vi "LED Loop.vi"   [LabVIEW 2016]
uses:
  <vilib>/Rock Robotics/WPI/DriverStation/WPI_DriverStationRobotMode2.ctl
  Common Code/Shooter Commands.ctl
  Robot Code/Robot Global Data.vi
types:
  T1 = typedef "Shooter Commands.ctl" = enum16{"Idle ", "Warmup ", "Shoot"}
  T2 = typedef "WPI_DriverStationRobotMode2.ctl" = enum16{"Autonomous Disabled", "Autonomous Enabled", "Teleop Disabled", "Teleop Enabled", "Disconnected", "Finish", "Test Disabled", "Test Enabled", "Emergency Stopped"}
  T3 = typedef "Shooter Control Cluster'.ctl" = cluster{"Shooter Modes":T4, "Shooter Commands":T1, "manUEL Control Cluster":T5, "Shot Type":T6}
  T4 = typedef "Shooter Modes.ctl" = enum16{"Auto", "Manual"}
  T5 = typedef "Manual Shoot Cluster.ctl" = cluster{"Shot RPM":dbl, "Wait Time":dbl, "da HOOD?":bool}
  T6 = typedef "Shot Type.ctl" = enum16{"Vision Shot", "Dist Shot", "Key Shot"}
  T7 = typedef "Climb Command Cluster.ctl" = cluster{"Go Up":bool}
  T8 = typedef "WPI_AOChannelDevRef.ctl" = cluster{"DevStatus":errorcluster, "AO Channel":T9}
  T9 = typedef "WPI_AnalogOutputChannel.ctl" = enum8{"AO MXP 0", "AO MXP 1", "Invalid"}
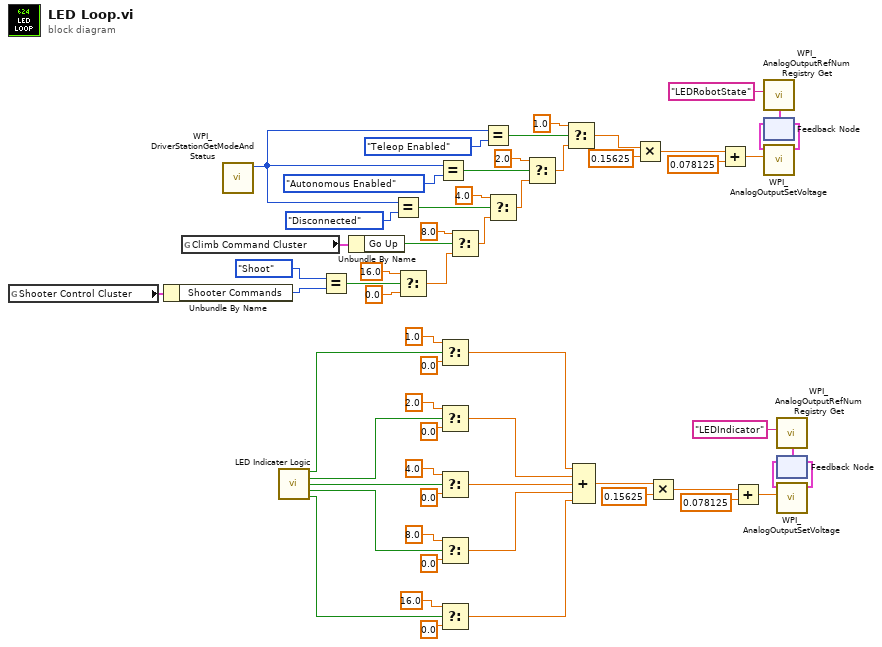
[diagram p0: block diagram]
diagram:
  n1 = global read "Robot Global Data.vi" "Shooter Control Cluster"() -> (w20:T3)
  n2 = Unbundle By Name(w20) -> ("Shooter Commands"=w18:T1)
  n3 = global read "Robot Global Data.vi" "Climb Command Cluster"() -> (w23:T7)
  n4 = call <vilib>:"WPI_DriverStationGetModeAndStatus.vi"() -> ("Robot Mode"=w27:T2)  [unwired: 10 in, 1 out]
  n5 = call "LED Indicater Logic.vi"() -> ("Read4Gear"=w61:bool, "Traction"=w58:bool, "Intake"=w57:bool, "Brakes"=w59:bool, "Hood Up"=w60:bool)  [unwired: 11 in]
  n6 = Equal?(x=Shooter_Commands."Shoot" ("Shooter Commands"), y=w18) -> (x = y?=w16:bool)
  n7 = Unbundle By Name(w23) -> ("Go Up"=w21:bool)
  n8 = Equal?(x=w27, y=WPI_DriverStationRobotMode2."Disconnected" ("Robot Mode")) -> (x = y?=w30:bool)
  n9 = Select(t=16.0, s=w16, f=0.0) -> (s? t:f=w17:dbl)
  n10 = Equal?(x=w27, y=WPI_DriverStationRobotMode2."Autonomous Enabled" ("Robot Mode")) -> (x = y?=w29:bool)
  n11 = Select(t=1.0, s=w61, f=0.0) -> (s? t:f=w46:dbl)
  n12 = Select(t=2.0, s=w58, f=0.0) -> (s? t:f=w45:dbl)
  n13 = Select(t=4.0, s=w57, f=0.0) -> (s? t:f=w44:dbl)
  n14 = Select(t=8.0, s=w59, f=0.0) -> (s? t:f=w43:dbl)
  n15 = Select(t=16.0, s=w60, f=0.0) -> (s? t:f=w42:dbl)
  n16 = Select(t=8.0, s=w21, f=w17) -> (s? t:f=w22:dbl)
  n17 = Equal?(x=w27, y=WPI_DriverStationRobotMode2."Teleop Enabled" ("Robot Mode")) -> (x = y?=w28:bool)
  n18 = Select(t=4.0, s=w30, f=w22) -> (s? t:f=w32:dbl)
  n19 = Select(t=2.0, s=w29, f=w32) -> (s? t:f=w31:dbl)
  n20 = Select(t=1.0, s=w28, f=w31) -> (s? t:f=w6:dbl)
  n21 = Compound Arithmetic op=ADD(w46, w45, w44, w43, w42) -> (w41:dbl)
  n22 = Multiply(x=w6, y=0.15625) -> (x*y=w8:dbl)
  n23 = Multiply(x=w41, y=0.15625) -> (x*y=w39:dbl)
  n24 = Add(x=w8, y=0.078125) -> (x+y=w1:dbl)
  n25 = Add(x=w39, y=0.078125) -> (x+y=w34:dbl)
  n26 = call <vilib>:"WPI_AnalogOutputRefNum Registry Get.vi"("refnum name"="LEDRobotState") -> ("AODeviceRef"=w4:T8)  [unwired: 9 in, 1 out]
  n27 = feedback #1(w4) -> (w3:T8)
  n28 = call <vilib>:"WPI_AnalogOutputSetVoltage.vi"("Voltage"=w1, "AODeviceRef"=w3) -> ("AODeviceRef"=w2:T8)  [unwired: 8 in, 1 out]
  n29 = feedback-in #1(w2) -> ()
  n30 = call <vilib>:"WPI_AnalogOutputRefNum Registry Get.vi"("refnum name"="LEDIndicator") -> ("AODeviceRef"=w35:T8)  [unwired: 9 in, 1 out]
  n31 = feedback #2(w35) -> (w36:T8)
  n32 = call <vilib>:"WPI_AnalogOutputSetVoltage.vi"("Voltage"=w34, "AODeviceRef"=w36) -> ("AODeviceRef"=w37:T8)  [unwired: 8 in, 1 out]
  n33 = feedback-in #2(w37) -> ()
